vi "Arduino.vi"() -> ()   [LabVIEW 2019]
uses:
  <vilib>/Instr/_visa.llb/VISA Configure Serial Port (Instr).vi
panel:
  out "Available?":bool
  in  "COM Port":refnum<visa-resource-name>
  in  "Baud Rate":u32=9600
  out "Num Inds":dbl
  in  "Stop Button":bool
  in  "Turn Off":bool
  in  "Turn On":bool
  out "Waveform Chart":dbl(graph)
  # "LM35"
  # "USB Control"
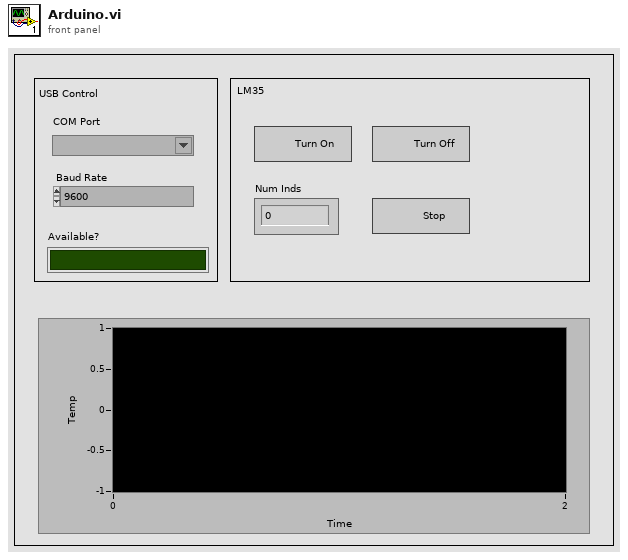
[diagram p1: front panel]
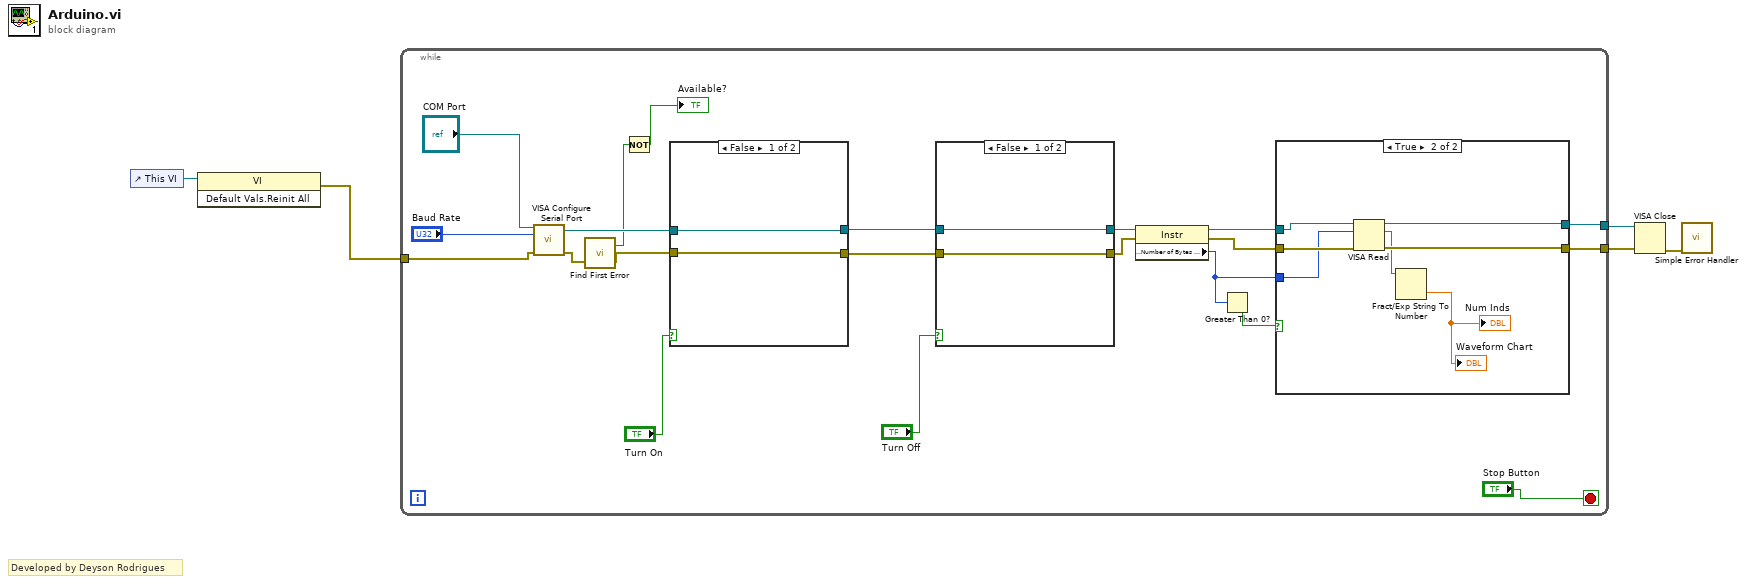
[diagram p0: block diagram]
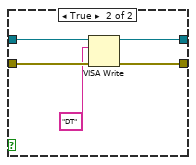
[diagram p3: hidden frame]
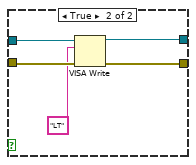
[diagram p4: hidden frame]
diagram:
  # "Developed by Deyson Rodrigues"
  n1 = control-ref of="This VI"() -> (w1:refnum<vi>)
  n2 = invoke class="VI" method="Default Vals.Reinit All"(reference=w1) -> (error out=w2:errorcluster)  [unwired: 2 in, 2 out]
  n3 = while {
    tunnel: [w19] -> w4
    tunnel: [w18] -> w5
    tunnel: w2 -> [w6]
    stop <- "Stop Button" stop-if-true
    n4 = call-poly "VISA Configure Serial Port"("VISA resource name"="COM Port", "baud rate (9600)"="Baud Rate", "error in (no error)"=w6) -> ("VISA resource name out"=w11:refnum<visa-resource-name>, "error out"=w9:errorcluster)  [unwired: 11 in]
    n5 = call <vilib>:"Find First Error.vi"("error in (no error)"=w9) -> ("error out"=w10:errorcluster, "error?"=w8:bool)  [unwired: 3 in]
    n6 = Not(x=w8) -> (.not. x?=→"Available?":bool)
    n7 = case shown="False" "Turn On" {
      tunnel: [w44 w49] -> w26
      tunnel: [w43 w48] -> w25
      tunnel: w11 -> [w44 w47]
      tunnel: w10 -> [w43 w46]
      frame False {
      }
      frame True {
        n8 = VISA Write(VISA resource name=w47, write buffer="LT", error in (no error)=w46) -> (VISA resource name out=w49:refnum<visa-resource-name>, error out=w48:errorcluster)  [unwired: 1 out]
      }
    }
    n9 = case shown="False" "Turn Off" {
      tunnel: w26 -> [w37 w42]
      tunnel: w25 -> [w36 w41]
      tunnel: [w36 w40] -> w23
      tunnel: [w37 w39] -> w24
      frame False {
      }
      frame True {
        n10 = VISA Write(VISA resource name=w42, write buffer="DT", error in (no error)=w41) -> (VISA resource name out=w39:refnum<visa-resource-name>, error out=w40:errorcluster)  [unwired: 1 out]
      }
    }
    n11 = property class="Instr"(reference=w24, error in=w23) -> (reference out=w20:refnum<visa-resource-name>, error out=w21:errorcluster, "Serial Settings:Number of Bytes at Serial Port"=w17:u32)
    n12 = Greater Than 0?(x=w17) -> (x > 0?=w22:bool)
    n13 = case shown="True" w22 {
      tunnel: w20 -> [w28 w35]
      tunnel: w21 -> [w27 w33]
      tunnel: [w28 w34] -> w19
      tunnel: [w27 w32] -> w18
      tunnel: w17 -> [_ w31]
      frame False {
      }
      frame True {
        n14 = VISA Read(VISA resource name=w35, byte count=w31, error in (no error)=w33) -> (VISA resource name out=w34:refnum<visa-resource-name>, read buffer=w30:string, error out=w32:errorcluster)  [unwired: 1 out]
        n15 = Fract/Exp String To Number(string=w30) -> (number=→"Num Inds" →"Waveform Chart":dbl)  [unwired: 3 in, 1 out]
      }
    }
  }
  n16 = VISA Close(VISA resource name=w4, error in (no error)=w5) -> (error out=w3:errorcluster)
  n17 = call <vilib>:"Simple Error Handler.vi"("error in (no error)"=w3) -> ()  [unwired: 4 in, 5 out]
